vi "Joystick and Camera dynamic dispatch.vi"(6 "XYZTheta":dbl[](array[numeric])=[651.719792, 50.568616, 0.000282, -0.000206], 8 "Tray Path":path=path "D:/Gantry_General/Qualification Results/Exercise3/tray.txt", 9 "Motion in":refnum<class "Motion.lvclass">=refnum) -> (0 "Fiducial Mark Position":dbl[][](array[numeric]), 1 "Gantry":dbl[](array[numeric])=[669.9515249261433, 125.68874001426492, 52.422846123058, -0.00020201540090827432] format="%#_8g", 2 "Sum":dbl[](array[numeric])=[669.9515249261433, 125.68874001426492, 52.422846123058, -0.00020201540090827432] format="%#_8g", 3 "Motion out":refnum<class "Motion.lvclass">)   [LabVIEW 2016]
uses:
  Classes/Controller/Camera/Camera Folder/Machine Vision.ctl
  Classes/Controller/Motion/Motion Folder/Motion.lvclass
  Classes/Controller/Motion/A3200 Folder/A3200.lvclass
  <vilib>/Utility/file.llb/Read Delimited Spreadsheet (DBL).vi
  <vilib>/Utility/file.llb/Write Delimited Spreadsheet (DBL).vi
  Classes/Controller/Camera/Camera Folder/Camera.lvclass
panel:
  out "Fiducial 2":dbl[](array[numeric])
  out "Fiducial 1":dbl[](array[numeric])
  in  "Go Fiducial 2":bool
  in  "Go Fiducial 1":bool
  in  "Record 2":bool
  in  "Record 1":bool
  in  "Go 3":bool
  out "Waveform Graph":dbl[](graph)
  out "Array 2":dbl[](array[numeric])
  out "Array":dbl[](array[numeric])
  out "Numeric":dbl
  out "Image 2":T1(plugin-control)
  in  "Machine Vision 2":T2
  in  "interval":dbl=0.005
  in  "focus":bool
  in  "Go 2":bool
  in  "Z Go":bool
  in  "Position":dbl
  in  "Machine Vision":T2=enum."INTT Sensor Cross"
  in  "Go":bool
  in  "Joystick":bool=TRUE
  in  "Stop":bool
  out "Image":T1(plugin-control)
  out "Camera":dbl[](array[numeric])=[0.14073295891284943, -0.06428433209657669] format="%#_8g"
  # "Please select Focus before pressing start !!!!!!!!!!"
types:
  T1 = typedef "IMAQ Image.ctl" = refnum<image>
  T2 = typedef "Camera.lvclass/Machine Vision.ctl" = enum16{"None", "chip cross 2", "chip cross", "Focus", "INTT HDI Mark", "INTT Sensor Cross", "INTT Chip Corner", "HPK Silicon", "Circle", "tpcb_hole"}
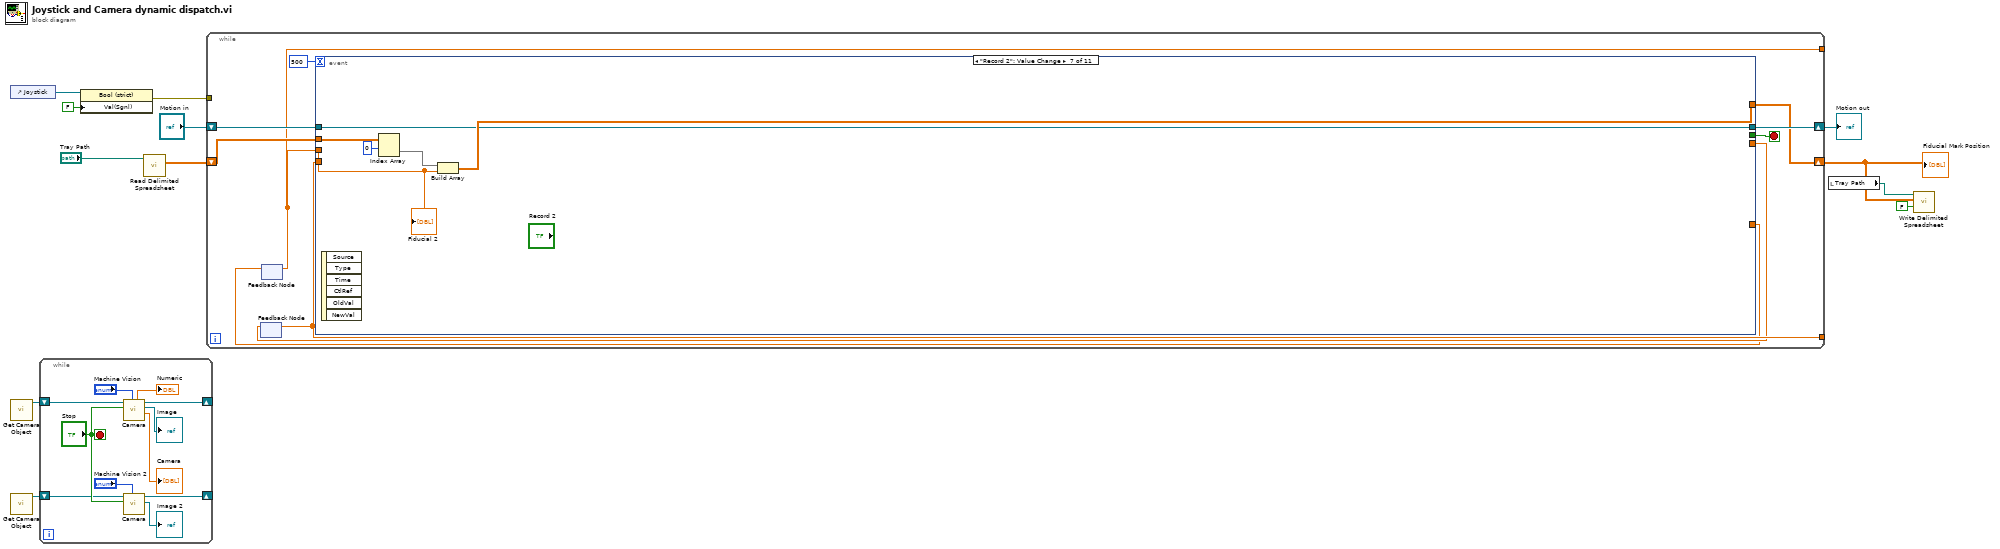
[diagram p0: block diagram]
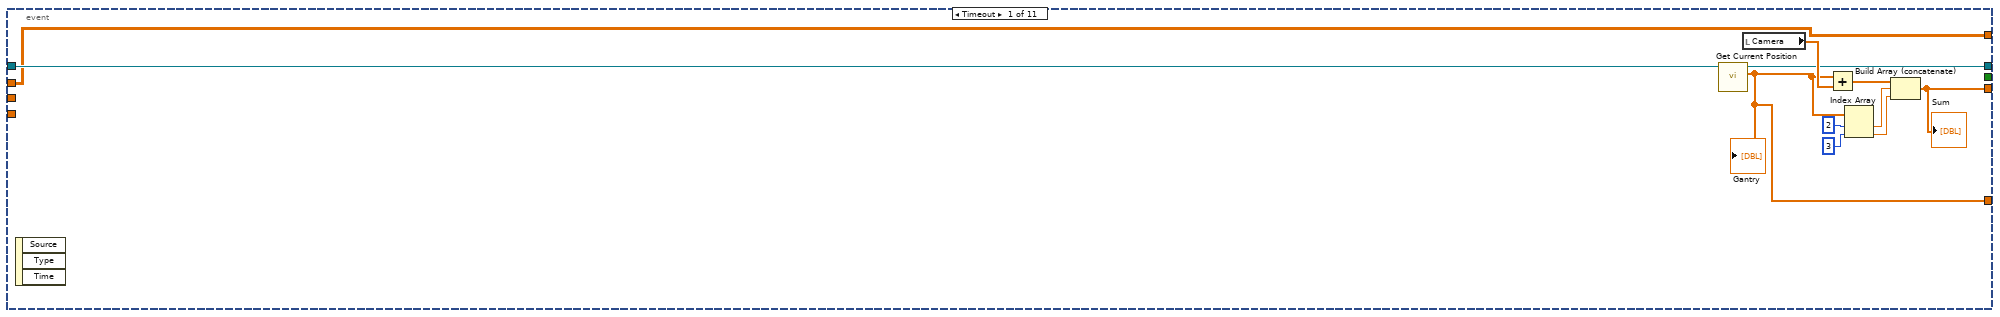
[diagram p2: hidden frame]
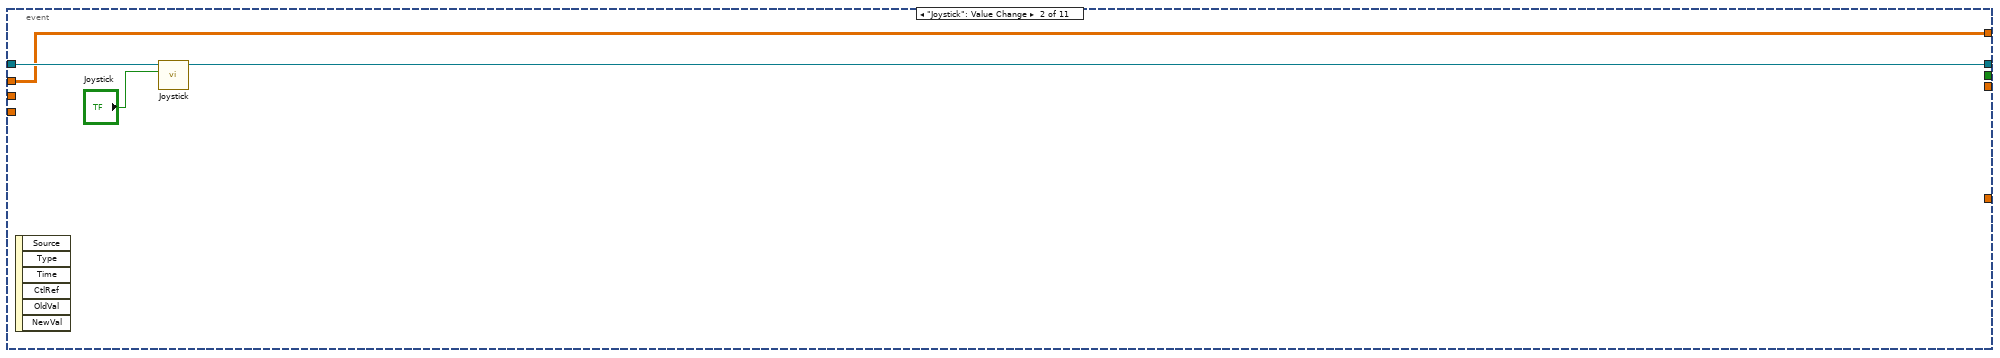
[diagram p3: hidden frame]
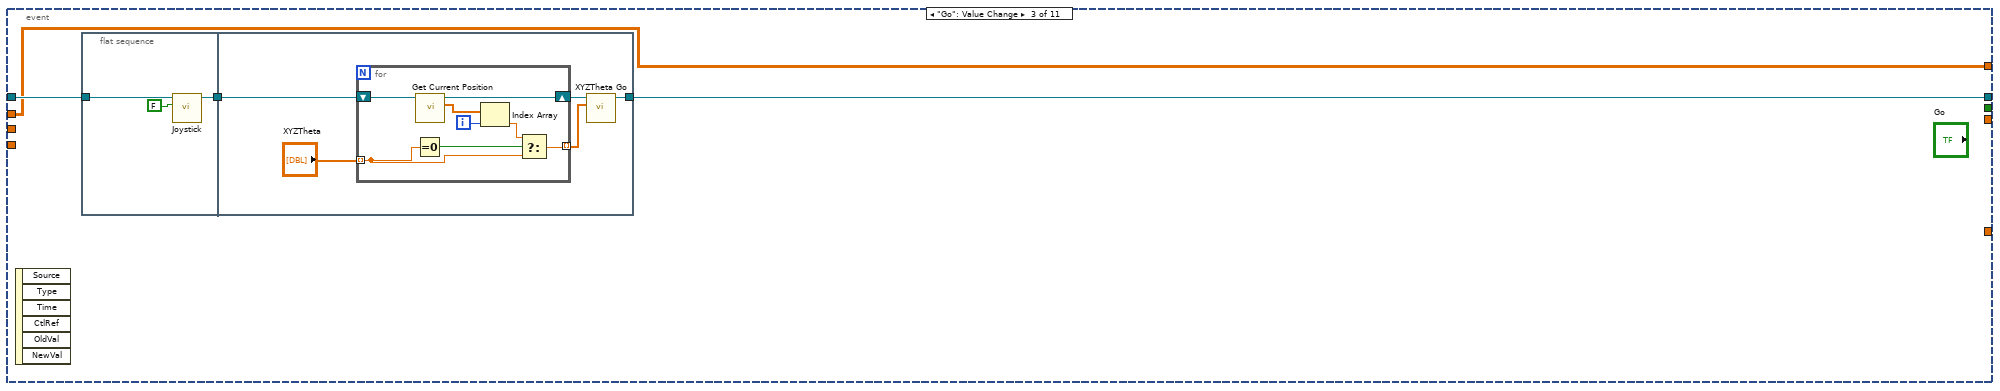
[diagram p4: hidden frame]
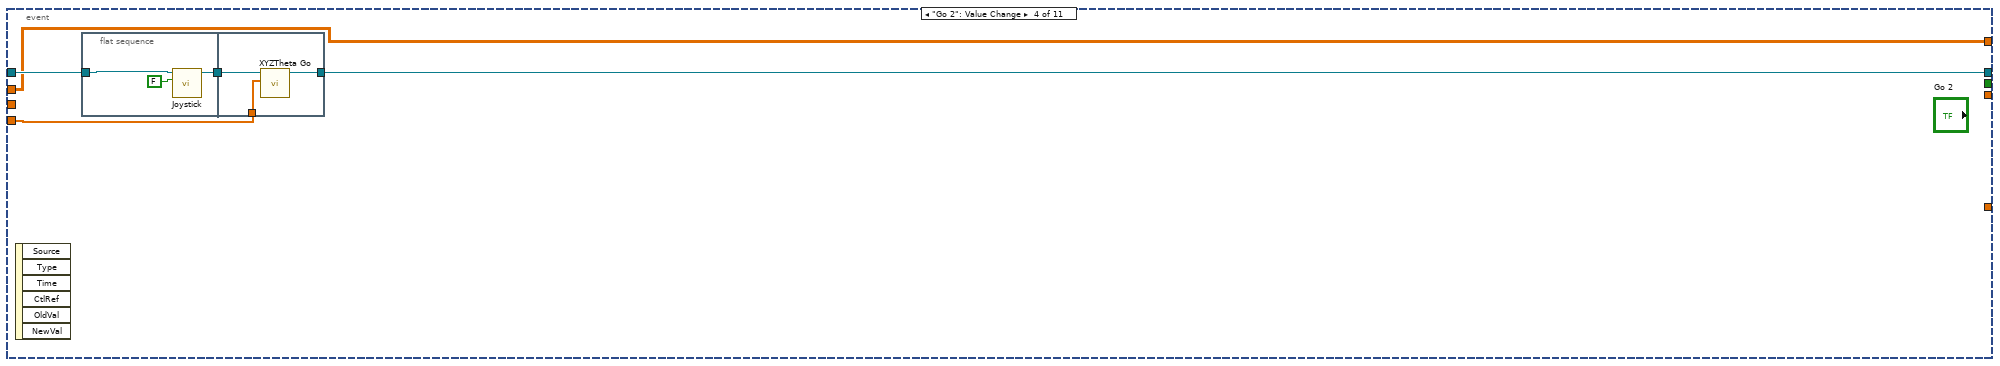
[diagram p5: hidden frame]
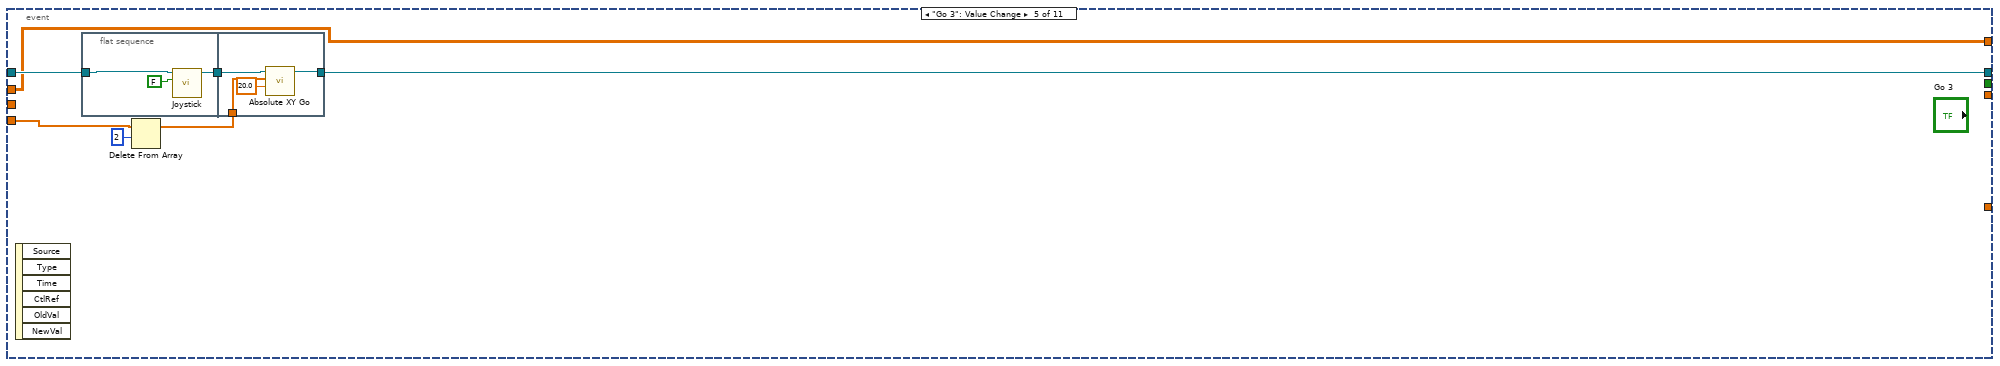
[diagram p6: hidden frame]
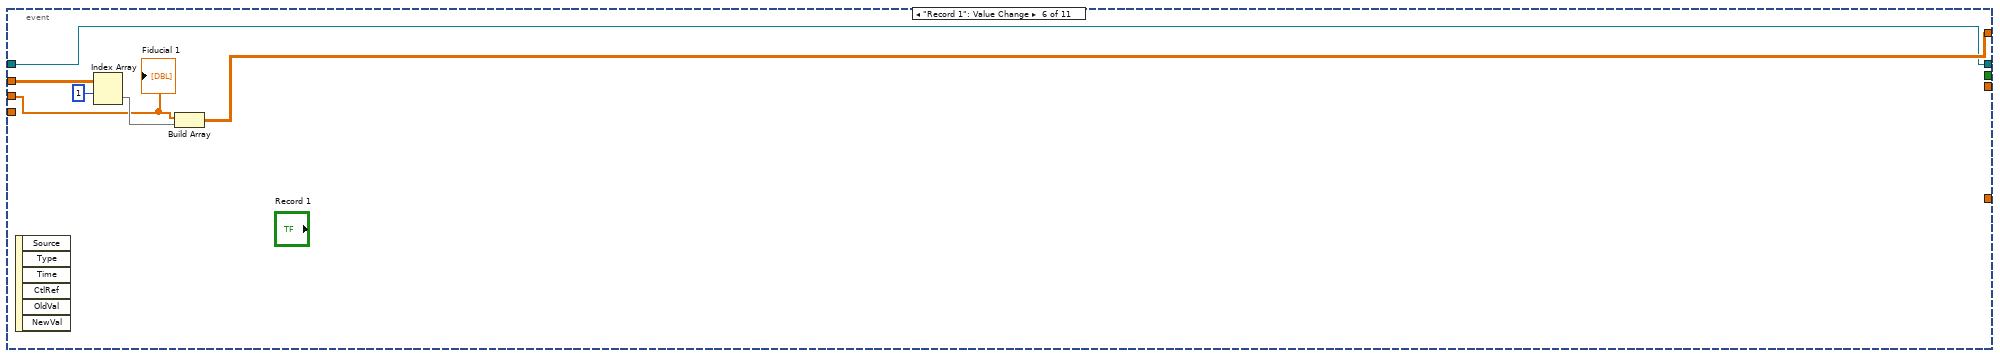
[diagram p7: hidden frame]
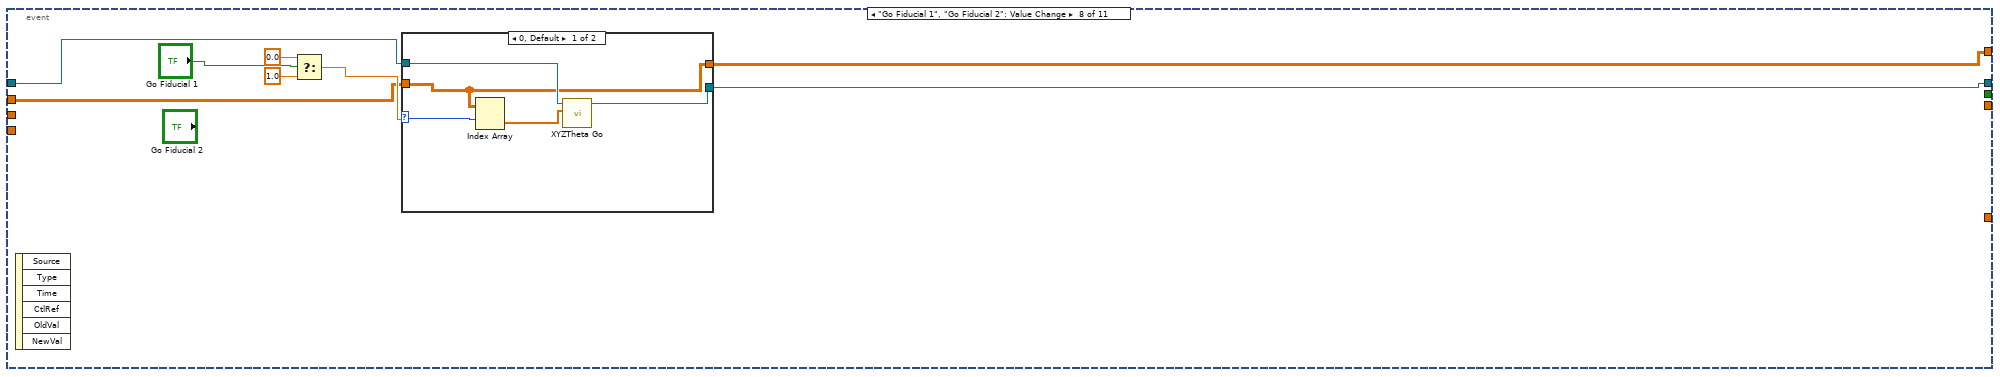
[diagram p8: hidden frame]
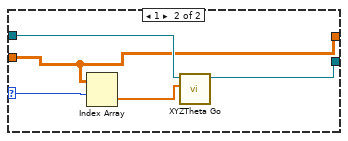
[diagram p9: hidden frame]
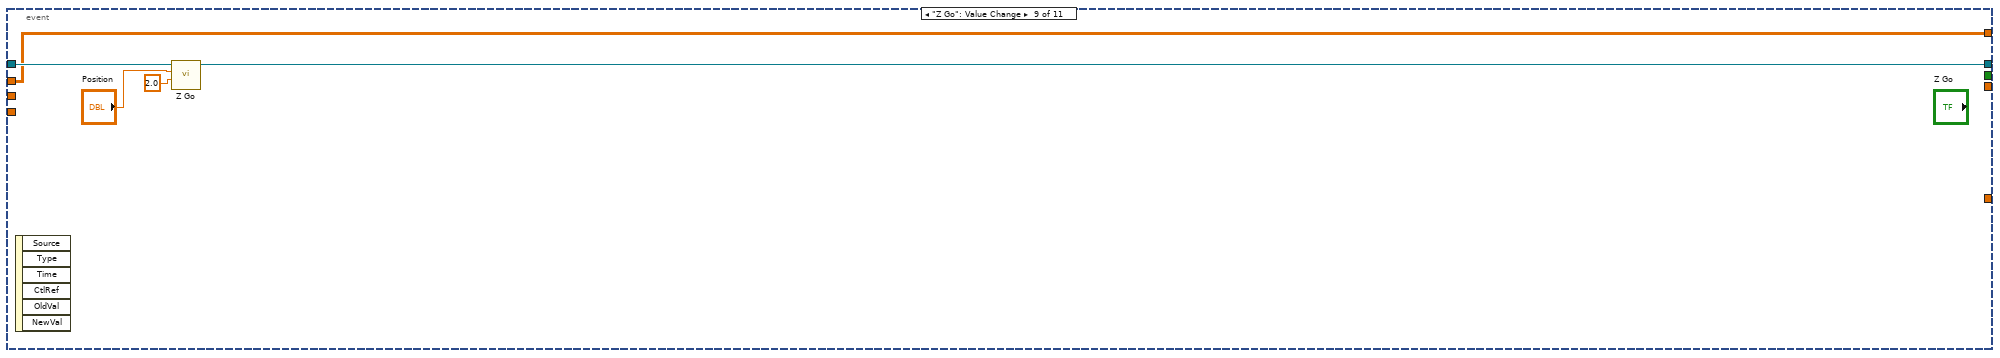
[diagram p10: hidden frame]
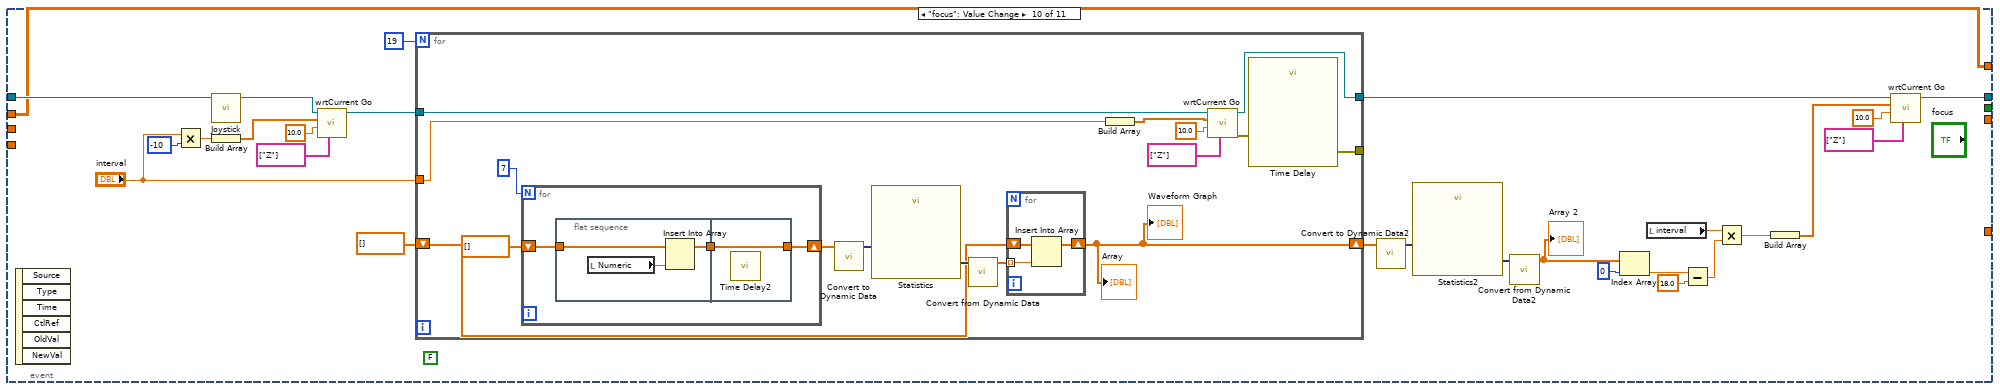
[diagram p11: hidden frame]
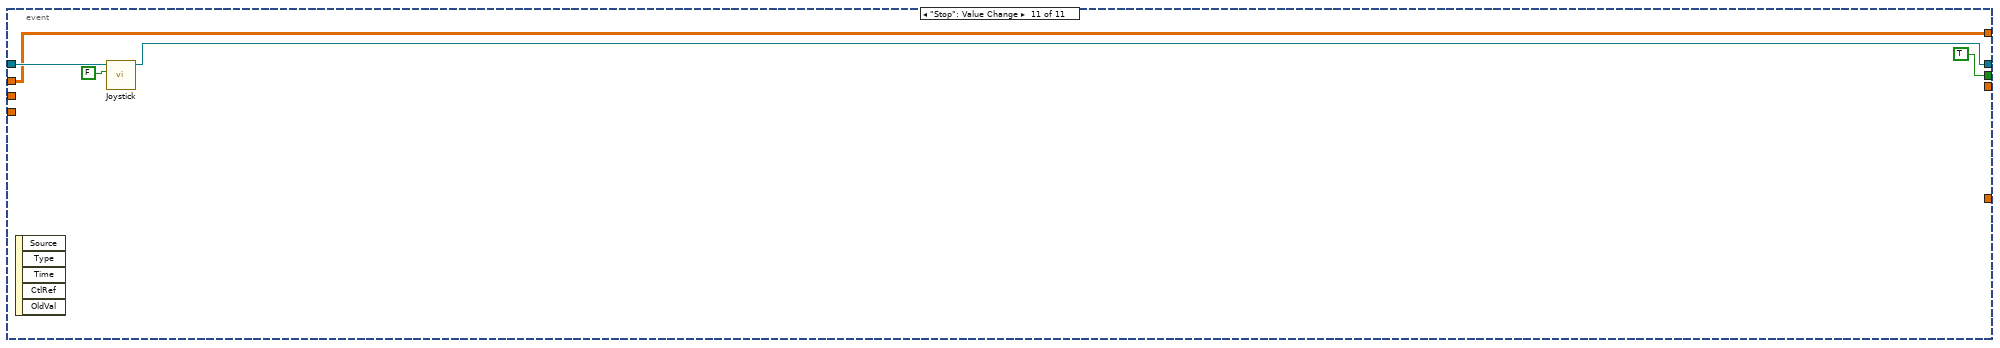
[diagram p12: hidden frame]
diagram:
  n1 = control-ref of="Joystick"() -> (w11:refnum<vi>)
  n2 = call "Get Camera Object.vi"() -> ("Camera out"=w9:refnum<class "Camera.lvclass">)  [unwired: 10 in, 1 out]
  n3 = call "Get Camera Object.vi"() -> ("Camera out"=w8:refnum<class "Camera.lvclass">)  [unwired: 10 in, 1 out]
  n4 = while {
    shift-right: [w22] -> _
    shift-left: w9 -> [w23]
    shift-right: [w15] -> _
    shift-left: w8 -> [w16]
    stop <- "Stop" stop-if-true
    n5 = call "Camera.vi"("Machine Vision"="Machine Vision", "Stop"="Stop", "Camera in"=w23) -> ("Camera"=→"Camera":dbl[], "Image"=→"Image":T1, "Camera out"=w22:refnum<class "Camera.lvclass">, "Numeric"=→"Numeric":dbl)  [unwired: 4 in, 1 out]
    n6 = call "Camera.vi"("Machine Vision"="Machine Vision 2", "Stop"="Stop", "Camera in"=w16) -> ("Image"=→"Image 2":T1, "Camera out"=w15:refnum<class "Camera.lvclass">)  [unwired: 4 in, 3 out]
  }
  n7 = property class="Bool (strict)"(reference=w11, "Val(Sgnl)"=FALSE ("Value (Signaling)")) -> (error out=w10:errorcluster)  [unwired: 1 in, 1 out]
  n8 = call-poly <vilib>:"Read Delimited Spreadsheet.vi"("file path (dialog if empty)"="Tray Path") -> ("all rows"=w4:dbl[][])  [unwired: 9 in, 5 out]
  n9 = while {
    shift-right: [w31] -> w6
    shift-left: "Motion in" -> [w28]
    tunnel: w10 -> [_]
    tunnel: [w30] -> _
    shift-right: [w26] -> w3
    shift-left: w4 -> [w27]
    tunnel: [w24] -> _
    stop <- w32 stop-if-true
    n10 = feedback #1() -> (w30:dbl[])  [unwired: 1 in]
    n11 = feedback #2() -> (w24:dbl[])  [unwired: 1 in]
    n12 = event shown="[6] \"Record 2\": Value Change" {
      selector: _ -> [_ _ _ _ _ _ _ _ _ _ _]
      dyn-events: _ -> [_ _ _ _ _ _ _ _ _ _ _]
      timeout: 500 -> [_ _ _ _ _ _ _ _ _ _ _]
      tunnel: [_ _ _ _ _ _ _ _ _ _ TRUE] -> w32
      tunnel: w28 -> [w43 w48 w52 w73 w86 w95 w101 w108 w128 w132 w185]
      tunnel: [w42 w46 w51 w72 w85 w95 w101 w107 w127 w140 w183] -> w31
      tunnel: [w39 _ _ _ _ _ _ _ _ _ _] -> w29
      tunnel: w30 -> [_ _ _ w70 w83 _ _ _ _ _ _]
      tunnel: w27 -> [w35 w45 w49 w69 w80 w99 w105 w109 w124 w129 w182]
      tunnel: [w35 w45 w49 w69 w80 w96 w103 w106 w124 w129 w182] -> w26
      tunnel: [w34 _ _ _ _ _ _ _ _ _ _] -> w25
      tunnel: w24 -> [_ _ _ _ _ w94 w100 _ _ _ _]
      event Timeout {
        n13 = event-data() -> ()  [unwired: 1 in, 3 out]
        n14 = call-dynamic "Get Current Position.vi"("Motion in"=w43) -> ("XYZTheta Out"=w34:dbl[], "Motion out"=w42:refnum<class "Motion.lvclass">)  [unwired: 8 in, 1 out]
        "Gantry" <- w34
        n15 = local read "Camera"() -> (w44:dbl[])
        n16 = Add(x=w34, y=w44) -> (x+y=w41:dbl[])
        n17 = Index Array(array=w34, index #1=2 ("index"), index #2=3 ("index")) -> (element #1=w37:dbl, element #2=w36:dbl)
        n18 = Build Array (concatenate)(w41, w37, w36) -> (w39:dbl[])
        "Sum" <- w39
      }
      event "Joystick": Value Change {
        n19 = event-data() -> ()  [unwired: 1 in, 6 out]
        n20 = call-dynamic "Joystick.vi"("Joystick"="Joystick", "Motion in"=w48) -> ("Motion out"=w46:refnum<class "Motion.lvclass">)  [unwired: 8 in, 1 out]
      }
      event "Go": Value Change {
        n21 = event-data() -> ()  [unwired: 1 in, 6 out]
        n22 = flat-sequence {
          tunnel: w52 -> [w54]
          tunnel: [w53] -> w50
          tunnel: [w56] -> w51
          tunnel: w50 -> [w59]
          frame #0 {
            n23 = call-dynamic "Joystick.vi"("Joystick"=FALSE, "Motion in"=w54) -> ("Motion out"=w53:refnum<class "Motion.lvclass">)  [unwired: 8 in, 1 out]
          }
          frame #1 {
            n24 = for {
              tunnel: "XYZTheta" -> [w66] mode=indexing
              tunnel: [w64] -> w58 mode=indexing
              shift-right: [w62] -> w57
              shift-left: w59 -> [w63]
              i -> [w68]
              n25 = Equal To 0?(x=w66) -> (x = 0?=w67:bool)
              n26 = call-dynamic "Get Current Position.vi"("Motion in"=w63) -> ("XYZTheta Out"=w61:dbl[], "Motion out"=w62:refnum<class "Motion.lvclass">)  [unwired: 8 in, 1 out]
              n27 = Index Array(array=w61, index=w68) -> (element=w65:dbl)
              n28 = Select(t=w65, s=w67, f=w66) -> (s? t:f=w64:dbl)
            }
            n29 = call "XYZTheta Go.vi"("XYZTheta In"=w58, "Motion in"=w57) -> ("Motion out"=w56:refnum<class "Motion.lvclass">)  [unwired: 7 in, 2 out]
          }
        }
      }
      event "Go 2": Value Change {
        n30 = event-data() -> ()  [unwired: 1 in, 6 out]
        n31 = flat-sequence {
          tunnel: w73 -> [w75]
          tunnel: [w74] -> w71
          tunnel: [w79] -> w72
          tunnel: w71 -> [w78]
          tunnel: w70 -> [w77]
          frame #0 {
            n32 = call-dynamic "Joystick.vi"("Joystick"=FALSE, "Motion in"=w75) -> ("Motion out"=w74:refnum<class "Motion.lvclass">)  [unwired: 8 in, 1 out]
          }
          frame #1 {
            n33 = call "XYZTheta Go.vi"("XYZTheta In"=w77, "Motion in"=w78) -> ("Motion out"=w79:refnum<class "Motion.lvclass">)  [unwired: 7 in, 2 out]
          }
        }
      }
      event "Go 3": Value Change {
        n34 = event-data() -> ()  [unwired: 1 in, 6 out]
        n35 = flat-sequence {
          tunnel: w86 -> [w88]
          tunnel: [w87] -> w84
          tunnel: [w90] -> w85
          tunnel: w84 -> [w91]
          tunnel: w81 -> [w93]
          frame #0 {
            n36 = call-dynamic "Joystick.vi"("Joystick"=FALSE, "Motion in"=w88) -> ("Motion out"=w87:refnum<class "Motion.lvclass">)  [unwired: 8 in, 1 out]
          }
          frame #1 {
            n37 = call-dynamic "Absolute XY Go.vi"("Speed"=20.0, "XY"=w93, "Motion in"=w91) -> ("Motion out"=w90:refnum<class "Motion.lvclass">)  [unwired: 7 in, 1 out]
          }
        }
        n38 = Delete From Array(array=w83, length=2) -> (array with subset deleted=w81:dbl[])  [unwired: 1 in, 1 out]
      }
      event "Record 1": Value Change {
        n39 = event-data() -> ()  [unwired: 1 in, 6 out]
        n40 = Index Array(array=w99, index (row)=1) -> (element=w97:dbl[])  [unwired: 1 in]
        n41 = Build Array(w94, w97) -> (w96:dbl[][])
        "Fiducial 1" <- w94
      }
      event "Record 2": Value Change {
        n42 = event-data() -> ()  [unwired: 1 in, 6 out]
        n43 = Index Array(array=w105, index (row)=0) -> (element=w102:dbl[])  [unwired: 1 in]
        n44 = Build Array(w102, w100) -> (w103:dbl[][])
        "Fiducial 2" <- w100
      }
      event "Go Fiducial 1", "Go Fiducial 2": Value Change {
        n45 = event-data() -> ()  [unwired: 1 in, 6 out]
        n46 = Select(t=0.0, s="Go Fiducial 1", f=1.0) -> (s? t:f=w110:dbl)
        n47 = case shown="0, Default" w110 {
          selector: w110 -> [w118 w123]
          tunnel: w109 -> [w114 w119]
          tunnel: w108 -> [w116 w121]
          tunnel: [w115 w120] -> w107
          tunnel: [w114 w119] -> w106
          frame 0, Default {
            n48 = Index Array(array=w114, index (row)=w118) -> (element=w117:dbl[])  [unwired: 1 in]
            n49 = call "XYZTheta Go.vi"("XYZTheta In"=w117, "Motion in"=w116) -> ("Motion out"=w115:refnum<class "Motion.lvclass">)  [unwired: 7 in, 2 out]
          }
          frame 1 {
            n50 = Index Array(array=w119, index (row)=w123) -> (element=w122:dbl[])  [unwired: 1 in]
            n51 = call "XYZTheta Go.vi"("XYZTheta In"=w122, "Motion in"=w121) -> ("Motion out"=w120:refnum<class "Motion.lvclass">)  [unwired: 7 in, 2 out]
          }
        }
      }
      event "Z Go": Value Change {
        n52 = event-data() -> ()  [unwired: 1 in, 6 out]
        n53 = call-dynamic "Z Go.vi"("Speed"=2.0, "Position"="Position", "Motion in"=w128) -> ("Motion out"=w127:refnum<class "Motion.lvclass">)  [unwired: 7 in, 1 out]
      }
      event "focus": Value Change {
        (unwired) FALSE ("Joystick")
        n54 = event-data() -> ()  [unwired: 1 in, 6 out]
        n55 = Multiply(x="interval", y=-10) -> (x*y=w148:dbl)
        n56 = call-dynamic "Joystick.vi"("Motion in"=w132) -> ("Motion out"=w131:refnum<class "Motion.lvclass">)  [unwired: 9 in, 1 out]
        n57 = Build Array(w148) -> (w150:dbl[])
        n58 = call-dynamic "wrtCurrent Go.vi"("Axis"=string[] ["Z"], "Speed"=10.0, "Distance"=w150, "Motion in"=w131) -> ("Motion out"=w154:refnum<class "Motion.lvclass">)  [unwired: 6 in, 1 out]
        n59 = for {
          N: 19 -> [_]
          tunnel: w154 -> [w156]
          tunnel: [w160] -> w139
          shift-right: [w157] -> w146
          shift-left: dbl[] [] -> [w158]
          tunnel: "interval" -> [w163]
          tunnel: [w159] -> _
          n60 = for {
            N: 7 -> [_]
            shift-right: [w177] -> w168
            shift-left: dbl[] [] -> [w176]
            n61 = flat-sequence {
              tunnel: w176 -> [w179]
              tunnel: [w180] -> w175
              tunnel: [w181] -> w177
              tunnel: w175 -> [w181]
              frame #0 {
                n62 = local read "Numeric"() -> (w178:dbl)
                n63 = Insert Into Array(array=w179, new element=w178) -> (w180:dbl[])  [unwired: 1 in]
              }
              frame #1 {
                n64 = call "Time Delay2"() -> ()  [unwired: 11 in, 1 out]
              }
            }
          }
          n65 = call "Convert to Dynamic Data"("Array"=w168) -> ("Dynamic Data Type"=w167:dynamicdata)  [unwired: 3 in]
          n66 = call "Statistics"("Signals"=w167) -> ("Arithmetic Mean"=w165:dynamicdata)  [unwired: 25 in, 1 out]
          n67 = call "Convert from Dynamic Data"("Dynamic Data Type"=w165) -> ("Array"=w161:dbl[])  [unwired: 3 in]
          n68 = for {
            tunnel: w161 -> [w174] mode=indexing
            shift-right: [w173] -> w157
            shift-left: w158 -> [w172]
            n69 = Insert Into Array(array=w172, new element=w174) -> (w173:dbl[])  [unwired: 1 in]
          }
          "Array" <- w157
          "Waveform Graph" <- w157
          n70 = Build Array(w163) -> (w162:dbl[])
          n71 = call-dynamic "wrtCurrent Go.vi"("Axis"=string[] ["Z"], "Speed"=10.0, "Distance"=w162, "Motion in"=w156) -> ("error out"=w169:errorcluster, "Motion out"=w160:refnum<class "Motion.lvclass">)  [unwired: 6 in]
          n72 = call "Time Delay"("error in (no error)"=w169) -> ("error out"=w159:errorcluster)  [unwired: 10 in]
        }
        n73 = call "Convert to Dynamic Data2"("Array"=w146) -> ("Dynamic Data Type"=w145:dynamicdata)  [unwired: 3 in]
        n74 = call "Statistics2"("Signals"=w145) -> ("Index of Max"=w144:dynamicdata)  [unwired: 25 in, 1 out]
        n75 = call "Convert from Dynamic Data2"("Dynamic Data Type"=w144) -> ("Array"=w130:dbl[])  [unwired: 3 in]
        "Array 2" <- w130
        n76 = Index Array(array=w130, index=0) -> (element=w134:dbl)
        n77 = local read "interval"() -> (w137:dbl)
        n78 = Subtract(x=w134, y=18.0 ("x")) -> (x-y=w138:dbl)
        n79 = Multiply(x=w137, y=w138) -> (x*y=w136:dbl)
        n80 = Build Array(w136) -> (w135:dbl[])
        n81 = call-dynamic "wrtCurrent Go.vi"("Axis"=string[] ["Z"], "Speed"=10.0, "Distance"=w135, "Motion in"=w139) -> ("Motion out"=w140:refnum<class "Motion.lvclass">)  [unwired: 6 in, 1 out]
      }
      event "Stop": Value Change {
        n82 = event-data() -> ()  [unwired: 1 in, 5 out]
        n83 = call-dynamic "Joystick.vi"("Joystick"=FALSE, "Motion in"=w185) -> ("Motion out"=w183:refnum<class "Motion.lvclass">)  [unwired: 8 in, 1 out]
      }
    }
    n84 = feedback-in #1(w29) -> ()
    n85 = feedback-in #2(w25) -> ()
  }
  "Motion out" <- w6
  "Fiducial Mark Position" <- w3
  n86 = local read "Tray Path"() -> (w1:path)
  n87 = call-poly <vilib>:"Write Delimited Spreadsheet.vi"("file path (dialog if empty)"=w1, "2D data"=w3, "append to file? (new file:F)"=FALSE) -> ()  [unwired: 11 in, 2 out]
